vi "Target.vi"() -> ()   [LabVIEW 2025]
uses:
  <vilib>/Platform/TimedLoop/XDataNode/timing_clust.ctl
  <vilib>/Platform/TimedLoop/XDataNode/nitl_modes.ctl
  <vilib>/Platform/TimedLoop/XDataNode/wakeup.ctl
  <vilib>/rvi/Emulation/niFpgaSctlEmulationGetInTimedLoop.vi
  <vilib>/rvi/Emulation/niFpgaEmulationReportErrorSimple.vi
  <vilib>/rvi/Emulation/niFpgaGetClockAttributes.vi
  <vilib>/rvi/Emulation/niFpgaCriticalErrorInLSC.vi
  <vilib>/rvi/linearAlgebra/MatrixMultiply/simVIs/SubVI/nifxpla_MatrixMultiply_SimMatrixSizes.vi
  <vilib>/rvi/linearAlgebra/MatrixMultiply/simVIs/SubVI/nifxpla_MatrixMultiply_Sim4WireAdapterVector.vi
  <vilib>/rvi/linearAlgebra/MatrixMultiply/simVIs/SubVI/nifxpla_MatrixMultiply_SimFrameHandShake.vi
  <vilib>/rvi/linearAlgebra/MatrixMultiply/simVIs/SubVI/nifxpla_MatrixMultiply_SimEndlessCounter.vi
  <vilib>/rvi/linearAlgebra/MatrixMultiply/simVIs/SubVI/nifxpla_MatrixMultiply_SimVectorDataBuffer.vi
  <vilib>/rvi/ClientSDK/Core/DevComputerLib/Private/Multiply(dfxp64).vi
  <vilib>/rvi/ClientSDK/Core/DevComputerLib/Private/Dfxp128ToDfxp256.vi
  <vilib>/rvi/ClientSDK/Core/DevComputerLib/Private/Add(dfxp256).vi
  <vilib>/rvi/ClientSDK/Core/DevComputerLib/Private/Subtract(dfxp256).vi
  <vilib>/rvi/ClientSDK/Core/DevComputerLib/Private/ToDfxp64(dfxp256).vi
  <vilib>/platform/TimedLoop/XDataNode/XDataNode.xnode
  <vilib>/rvi/linearAlgebra/MatrixMultiply/XNode/nifxpla_MatrixMultiply.xnode
  <vilib>/rvi/linearAlgebra/MatrixMultiply/simVIs/nifxpla_MatrixMultiply_SimTemplateEinEout.vi
  <vilib>/rvi/linearAlgebra/MatrixMultiply/simVIs/nifxpla_MatrixMultiply_SimTemplateEinVout.vi
  <vilib>/rvi/linearAlgebra/MatrixMultiply/simVIs/nifxpla_MatrixMultiply_SimTemplateVinEout.vi
  <vilib>/rvi/linearAlgebra/MatrixMultiply/simVIs/nifxpla_MatrixMultiply_SimTemplateVinVout.vi
  <vilib>/Platform/TimedLoop/XDataNode/XDNodeRunTimeDep.lvlib
panel:
  out "Array 3":bool[](array[boolean])
  out "Array 2":i32[](array[numeric])
  out "Array":bool[](array[boolean])
  out "C":fxp<+/-,32,16>[](array[numeric])
  out "Cycle Count":i32
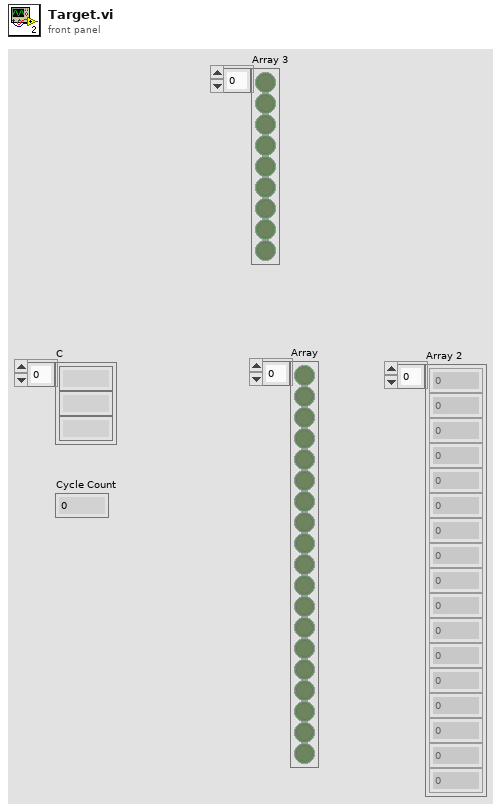
[diagram p1: front panel]
types:
  T1 = typedef "XDNodeRunTimeDep.lvlib/timing_clust.ctl" = cluster{"Expected End [f-1]":u64, "Actual End [f-1]":u64, "Finished Late? [f-1]":bool, "Expected End [i-1]":u64, "Actual End [i-1]":u64, "Finished Late? [i-1]":bool, "Expected Start [i]":u64, "Actual Start [i]":u64, "Expected Start [f]":u64, "Actual Start [f]":u64, "Source Name":string, "Structure Name":string, "Period":i64, "Deadline":i64, "Offset":i64, "Start":i64, "Priority":i32, "Timeout":i32, "Mode":T2, "Wakeup Reason":T3, "Error":errorcluster, "Source Type":string, "Secondary Source Type":string, "Global End Time":u64, "Global Start Time":u64, "Frame Duration":u64, "Iteration Duration":u64, "Assigned CPU":i32, "I/O Scan Engine Mode":u32}
  T2 = typedef "XDNodeRunTimeDep.lvlib/nitl_modes.ctl" = enum32{"No Change", "Process missed periods, maintain original phase", "Discard missed periods, maintain original phase", "Process missed periods, ignore original phase", "Discard missed periods, ignore original phase"}
  T3 = typedef "XDNodeRunTimeDep.lvlib/wakeup.ctl" = enum32{"Normal", "Aborted", "Asynchronous wakeup", "Timing source error", "Timed loop error", "Timeout"}
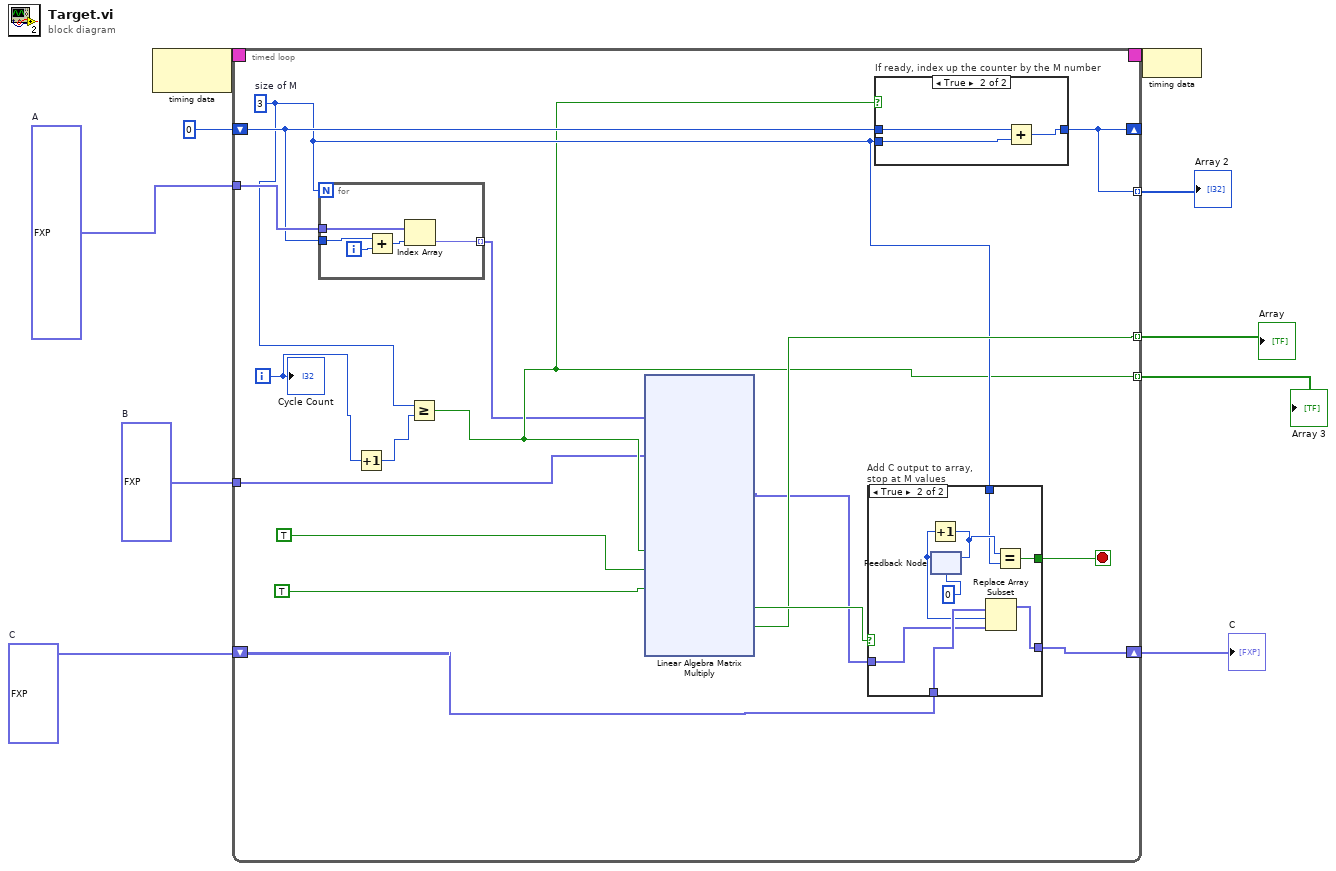
[diagram p0: block diagram]
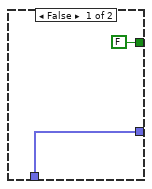
[diagram p3: hidden frame]
diagram:
  w6 = fxp<+/-,32,16>[] [1.0, 2.0, 3.0, 4.0, 5.0, 6.0, 7.0, 8.0, 9.0]  # A
  w7 = fxp<+/-,32,16>[] [1.0, 2.0, 3.0]  # B
  w8 = fxp<+/-,32,16>[] [0.0, 0.0, 0.0]  # C
  n1 = node-c288() -> (w10:T1)  [unwired: 1 in]
  n2 = timed-loop {
    timing: w10 -> [_]
    timing-out: [_] -> w9
    shift-right: [w25] -> w5
    shift-left: w8 -> [w24]
    tunnel: w7 -> [w12]
    tunnel: w6 -> [w22]
    shift-right: [w18] -> _
    shift-left: 0 ("length") -> [w21]
    tunnel: [w19] -> w3 mode=indexing
    tunnel: [w18] -> w2 mode=indexing
    tunnel: [w16] -> w1 mode=indexing
    i -> [w15]
    stop <- w23 stop-if-true
    w17 = 3  # size of M
    n3 = for {
      N: w17 -> [_]
      tunnel: w22 -> [w32]
      tunnel: w21 -> [w30]
      tunnel: [w28] -> w13 mode=indexing
      i -> [w31]
      n4 = Add(x=w30, y=w31) -> (x+y=w29:i32)
      n5 = Index Array "Index Array"(array=w32, index=w29) -> (element=w28:fxp<+/-,32,16>)
    }
    n6 = Increment(x=w15) -> (x+1=w14:i32)
    n7 = Greater Or Equal?(x=w17, y=w14) -> (x >= y?=w16:bool)
    n8 = xnode ("Linear Algebra Matrix Multiply")("ar"=w13, "br"=w12, "a valid"=w16, "b valid"=TRUE, "ready for output (T)"=TRUE) -> ("cr"=w11:fxp<+/-,32,16>[], "output valid"=w26:bool, "ready for a"=w19:bool)  [unwired: 2 in, 3 out]
    n9 = case "Add C output to array, stop at M values" shown="True" w26 {
      tunnel: w11 -> [_ w42]
      tunnel: [w38 w45] -> w25
      tunnel: w24 -> [w38 w46]
      tunnel: [FALSE w43] -> w23
      tunnel: w17 -> [_ w39]
      frame False {
      }
      frame True {
        n10 = feedback #1(0 ("x")) -> (w41:i32)
        n11 = Increment(x=w41) -> (x+1=w40:i32)
        n12 = feedback-in #1(w40) -> ()
        n13 = Replace Array Subset(array=w46, new element=w42, index=w41) -> (w45:fxp<+/-,32,16>[])
        n14 = Equal?(x=w40, y=w39) -> (x = y?=w43:bool)
      }
    }
    n15 = case "If ready, index up the counter by the M number" shown="True" w16 {
      tunnel: w21 -> [w33 w36]
      tunnel: [w33 w35] -> w18
      tunnel: w17 -> [_ w34]
      frame False {
      }
      frame True {
        n16 = Add(x=w36, y=w34) -> (x+y=w35:i32)
      }
    }
    "Cycle Count" <- w15
  }
  "C" <- w5
  "Array" <- w3
  "Array 2" <- w2
  "Array 3" <- w1
  n17 = node-c288(w9) -> ()
